vi "ComputeRectAverage_Depth.vi"(5 "Error In":errorcluster, 6 "Image Pixels (U8)":u8[][](array[numeric])) -> (0 "error IO":errorcluster, 3 "Davg":dbl)   [LabVIEW 2012]
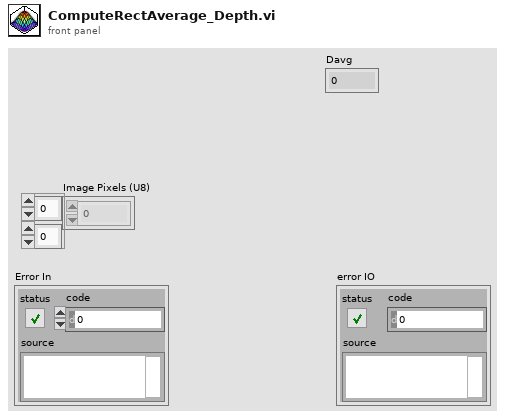
[diagram p1: front panel]
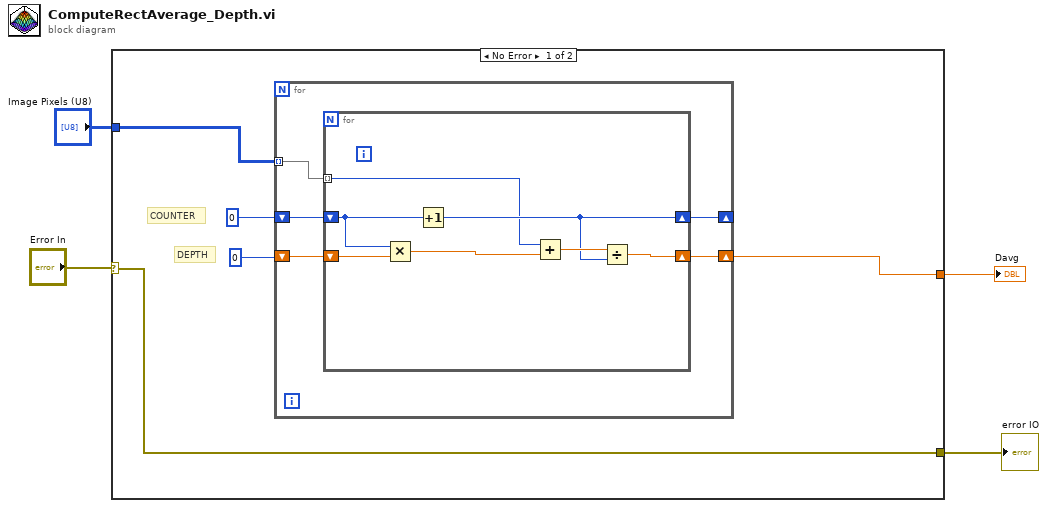
[diagram p0: block diagram]
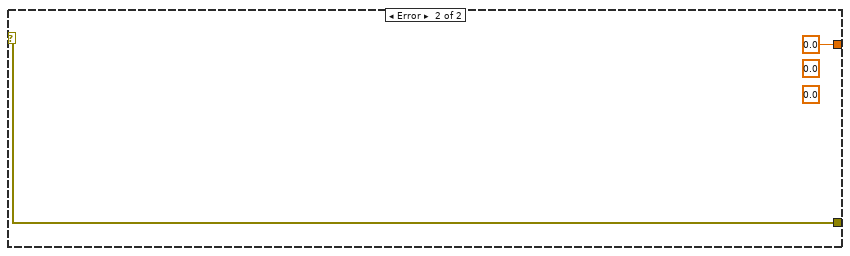
[diagram p2: hidden frame]
diagram:
  n1 = case shown="No Error" "Error In" {
    selector: "Error In" -> [w8 w23]
    tunnel: [w8 w23] -> w3
    tunnel: "Image Pixels (U8)" -> [w7 _]
    tunnel: [w5 0.0] -> w1
    frame No Error {
      # "COUNTER"
      # "DEPTH"
      n2 = for {
        tunnel: w7 -> [w14] mode=indexing
        shift-right: [w12] -> w5
        shift-left: u16 0 -> [w13]
        shift-right: [w10] -> _
        shift-left: u64 0 -> [w11]
        n3 = for {
          tunnel: w14 -> [w15] mode=indexing
          shift-right: [w18] -> w12
          shift-left: w13 -> [w21]
          shift-right: [w16] -> w10
          shift-left: w11 -> [w17]
          n4 = Multiply(x=w17, y=w21) -> (x*y=w20:dbl)
          n5 = Increment(x=w17) -> (x+1=w16:u64)
          n6 = Add(x=w15, y=w20) -> (x+y=w19:dbl)
          n7 = Divide(x=w19, y=w16) -> (x/y=w18:dbl)
        }
      }
    }
    frame Error {
      (unwired) 0.0
      (unwired) 0.0
    }
  }
  "error IO" <- w3
  "Davg" <- w1
